vi "create sql query SRS delays expt editor scan start and end.vi"(10 "exptdeviceID":string="xxx", 11 "Expt editor SCS on":T1 {"Scan End" format="%#_6p"; "Scan Start" format="%#_6p"}) -> (3 "Array":string[](array[string]))   [LabVIEW 2020]
uses:
  experiment editor scan delays SCS on off.ctl
  delay scan start and end.ctl
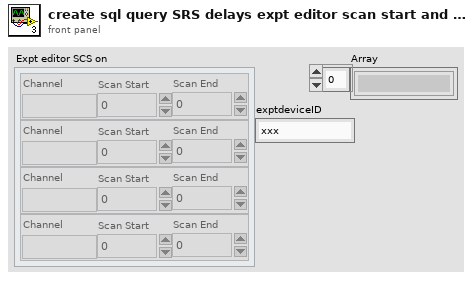
[diagram p1: front panel]
types:
  T1 = typedef "experiment editor scan delays SCS on off.ctl" = T2[]
  T2 = typedef "delay scan start and end.ctl" = cluster{"Channel":string, "Scan Start":dbl, "Scan End":dbl}
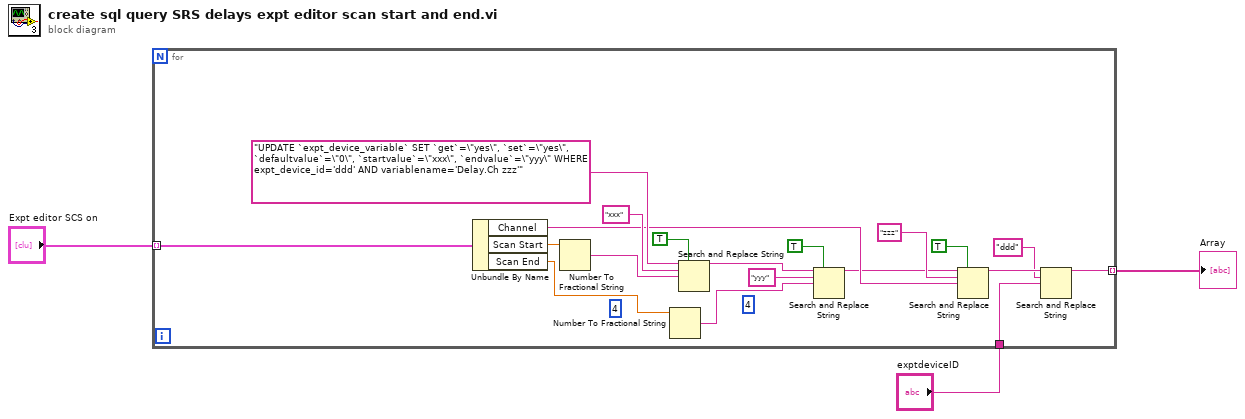
[diagram p0: block diagram]
diagram:
  n1 = for {
    tunnel: "Expt editor SCS on" -> [w18] mode=indexing
    tunnel: [w6] -> w3 mode=indexing
    tunnel: "exptdeviceID" -> [w4]
    (unwired) i16 4 ("precision (6)")
    (unwired) i16 4 ("precision (6)")
    n2 = Unbundle By Name(w18) -> ("Channel"=w9:string, "Scan Start"=w17:dbl, "Scan End"=w12:dbl)
    n3 = Number To Fractional String(number=w17) -> (F-format string=w19:string)  [unwired: 3 in]
    n4 = Number To Fractional String(number=w12) -> (F-format string=w16:string)  [unwired: 3 in]
    n5 = Search and Replace String(replace all?=TRUE ("replace all? (F)"), input string="UPDATE `expt_device_variable` SET `get`=\"yes\", `set`=\"yes\", `defaultvalue`=\"0\", `startvalue`=\"xxx\", `endvalue`=\"yyy\" WHERE expt_device_id='ddd' AND variablename='Delay.Ch zzz'" ("Query"), search string="xxx", replace string=w19) -> (result string=w13:string)  [unwired: 4 in, 3 out]
    n6 = Search and Replace String(replace all?=TRUE ("replace all? (F)"), input string=w13, search string="yyy", replace string=w16) -> (result string=w8:string)  [unwired: 4 in, 3 out]
    n7 = Search and Replace String(replace all?=TRUE ("replace all? (F)"), input string=w8, search string="zzz", replace string=w9) -> (result string=w7:string)  [unwired: 4 in, 3 out]
    n8 = Search and Replace String(input string=w7, search string="ddd", replace string=w4) -> (result string=w6:string)  [unwired: 5 in, 3 out]
  }
  "Array" <- w3
